vi "6_3_2.vi"(11 "VI (Eingang)":refnum<vi>) -> (3 "Map":map{string, refnum<vi>}(c390))   [LabVIEW 2020]
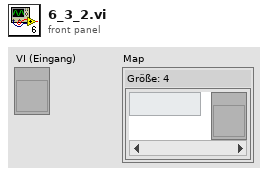
[diagram p1: front panel]
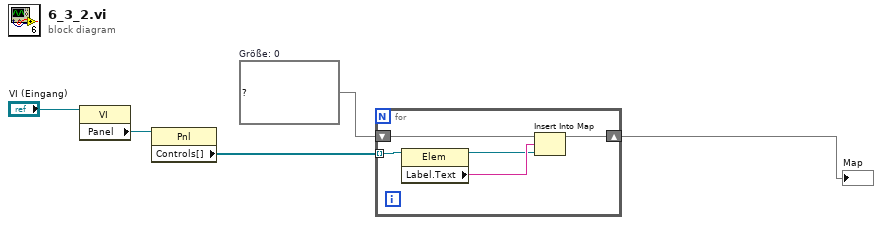
[diagram p0: block diagram]
diagram:
  w3 = map{string, refnum<vi>} {}  # Größe: 0
  n1 = property class="VI"(reference="VI (Eingang)") -> ("Panel"=w2:refnum<vi>)  [unwired: 1 in, 2 out]
  n2 = property class="Pnl"(reference=w2) -> ("Controls[]"=w5:refnum<vi>[])  [unwired: 1 in, 2 out]
  n3 = for {
    tunnel: w5 -> [w10] mode=indexing
    shift-right: [w6] -> w4
    shift-left: w3 -> [w7]
    n4 = property class="Elem"(reference=w10) -> (reference out=w8:refnum<vi>, "Label.Text"=w9:string)  [unwired: 1 in, 1 out]
    n5 = Insert Into Map(map in=w7, key=w9, value=w8) -> (map out=w6:map{string, refnum<vi>})  [unwired: 2 out]
  }
  "Map" <- w4
